vi "Change Tag Select Name.vi"(6 "Variant":variant, 8 "error in (no error)":errorcluster, 9 "old values":string[][](array[string]), 10 "object ref in":T1, 11 "Cluster":T2) -> (0 "error out":errorcluster)   [LabVIEW 2015, in "tag select module editor node.lvclass"]
uses:
  tag select module editor node.lvclass
  <vilib>/NI/DCAF/Tag Editor Core/Table API/Table Manager/Cell Change.ctl
  <vilib>/NI/DCAF/Tag Editor Core/Table API/Table Manager/object ref.ctl
  <vilib>/NI/DCAF/Tag Editor Core/Configuration Editor/Classes/Engine Parent/Engine Parent Editor Node.lvclass
  <vilib>/NI/DCAF/Tag Editor Core/Configuration Editor/Classes/Module editor node/module editor node.lvclass
  module/configuration/tag select module configuration.lvclass
  module/configuration/tag select module configuration.lvclass/tag select module configuration.ctl
  <vilib>/NI/DCAF/Tag Editor Core/Table API/Table Manager.lvlib
  <vilib>/NI/DCAF/Tag Editor Core/Table API/Table Manager/Table Manager.lvclass
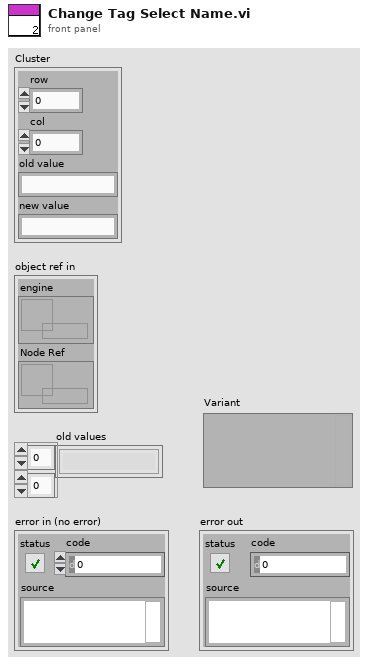
[diagram p1: front panel]
types:
  T1 = typedef "Table Manager.lvlib/Table Manager.lvclass/object ref.ctl" = cluster{"engine":refnum<data-value>, "Node Ref":refnum<data-value>}
  T2 = typedef "Table Manager.lvlib/Cell Change.ctl" = cluster{"row":i32, "col":i32, "old value":string, "new value":string}
  T3 = typedef "tag select module configuration.lvclass/tag select configuration.ctl" = cluster{"tag select name":string, "data type":T4, "output":refnum<class "TBM channel.lvclass">, "select":refnum<class "TBM channel.lvclass">, "input channels":refnum<class "TBM channel.lvclass">[]}
  T4 = typedef "tag bus.lvlib/tag descriptor.lvclass/Data Type.ctl" = enum16{"Double", "Single", "I64", "I32", "I16", "I8", "U64", "U32", "U16", "U8", "Boolean", "String", "Array of Double", "Array of Single", "Array of I64", "Array of I32", "Array of I16", "Array of I8", "Array of U64", "Array of U32", "Array of U16", "Array of U8", "Array of Boolean", "Array of String"}
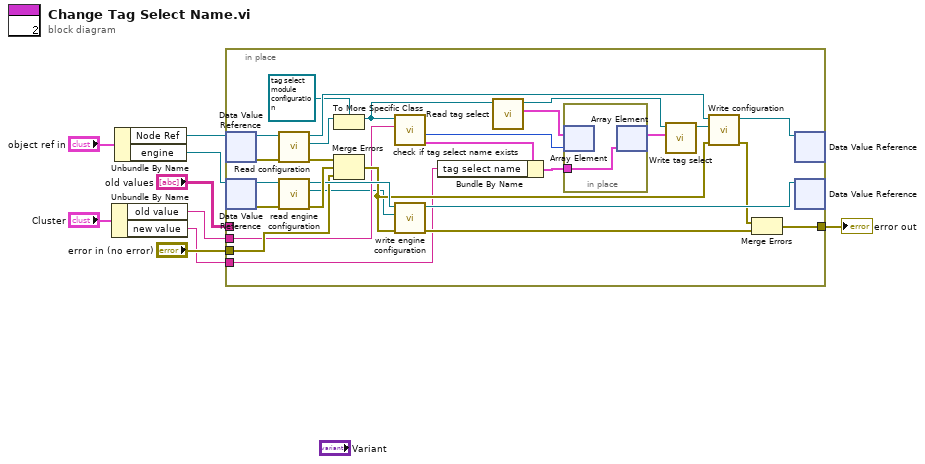
[diagram p0: block diagram]
diagram:
  n1 = Unbundle By Name("Cluster") -> ("old value"=w2:string, "new value"=w1:string)
  n2 = Unbundle By Name("object ref in") -> ("Node Ref"=w4:refnum<data-value>, "engine"=w3:refnum<data-value>)
  n3 = in-place {
    in-place-border: [w29] -> w8
    in-place-border: "error in (no error)" -> [w21]
    in-place-border: "old values" -> [_]
    in-place-border: w2 -> [w14]
    in-place-border: w1 -> [w13]
    n4 = in-place-dvr #1(w4) -> (w26:refnum<class "module editor node.lvclass">, w28:errorcluster)
    n5 = in-place-dvr #2(w3) -> (w36:refnum<class "Engine Parent Editor Node.lvclass">, w37:errorcluster)
    n6 = call-dynamic "Read configuration.vi"("error in"=w28, "NISE_CEF_serializable node in"=w26) -> ("error out"=w27:errorcluster, "configuration"=w24:refnum<class "NISE_CEF_serializable configuration.lvclass">, "NISE_CEF_serializable node out"=w25:refnum<class "module editor node.lvclass">)  [unwired: 7 in]
    n7 = call <vilib>:"read engine configuration.vi"("error in"=w37, "Engine Parent Editor Node in"=w36) -> ("error out"=w33:errorcluster, "engine configuration"=w10:refnum<class "engine configuration.lvclass">, "Engine Parent Editor Node out"=w32:refnum<class "Engine Parent Editor Node.lvclass">)  [unwired: 7 in]
    n8 = To More Specific Class(target class=refnum<class "tag select module configuration.lvclass"> refnum ("tag select module configuration"), reference=w24) -> (specific class reference=w20:refnum<class "tag select module configuration.lvclass">)  [unwired: 1 in, 1 out]
    n9 = Merge Errors(w27, w33, w21) -> (w23:errorcluster)
    n10 = call "check if tag select name exists.vi"("name to locate"=w14, "tag select module configuration in"=w20) -> ("tag select config"=w15:T3, "index"=w16:i32)  [unwired: 6 in, 2 out]
    n11 = call <vilib>:"write engine configuration.vi"("error in"=w23, "engine configuration"=w10, "Engine Parent Editor Node in"=w32) -> ("error out"=w31:errorcluster, "Engine Parent Editor Node out"=w35:refnum<class "Engine Parent Editor Node.lvclass">)  [unwired: 7 in]
    n12 = Bundle By Name(cluster=w15, "tag select name"=w13) -> (w12:T3)
    n13 = call "Read tag select.vi"("tag select module configuration in"=w20) -> ("tag select"=w19:T3[], "tag select module configuration out"=w17:refnum<class "tag select module configuration.lvclass">)  [unwired: 8 in, 1 out]
    n14 = in-place {
      in-place-border: w12 -> [w38]
      n15 = in-place-array #3(w19, w16) -> ()  [unwired: 1 out]
      n16 = in-place-array #3(w38) -> (w18:T3[])  [unwired: 1 out]
    }
    n17 = call "Write tag select.vi"("tag select"=w18, "tag select module configuration in"=w17) -> ("tag select module configuration out"=w11:refnum<class "tag select module configuration.lvclass">)  [unwired: 8 in, 1 out]
    n18 = call-dynamic "Write configuration.vi"("error in"=w23, "configuration"=w11, "NISE_CEF_serializable node in"=w25) -> ("error out"=w30:errorcluster, "NISE_CEF_serializable node out"=w34:refnum<class "module editor node.lvclass">)  [unwired: 7 in]
    n19 = Merge Errors(w30, w31) -> (w29:errorcluster)
    n20 = in-place-dvr #1(w34) -> ()  [unwired: 2 out]
    n21 = in-place-dvr #2(w35) -> ()  [unwired: 2 out]
  }
  "error out" <- w8
